vi "Quick Load WAV.vi"(8 "error in":errorcluster, 11 "Data":u8[](array[numeric])) -> (0 "error out":errorcluster, 3 "Chunk Pointer":u32 format="%.0x")   [LabVIEW 2014, in "LibSDL2_Mixer.lvlib"]
uses:
  LibSDL2_Mixer.lvlib
  LibSDL2 Wrapper/DLL/SDL2_mixer.dll
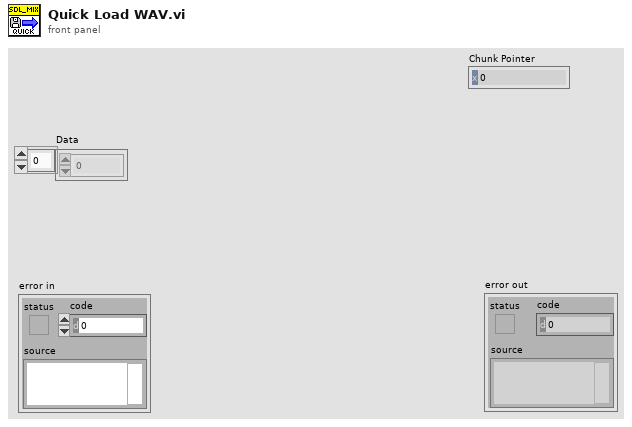
[diagram p1: front panel]
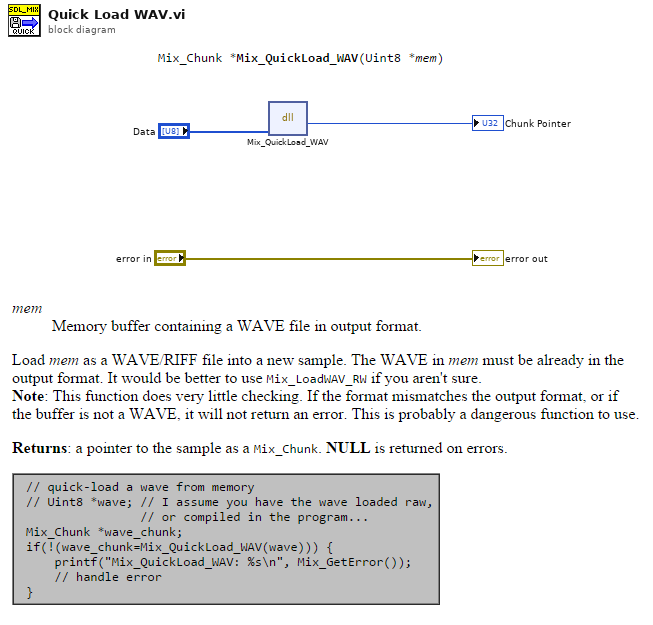
[diagram p0: block diagram]
diagram:
  n1 = dll-call lib="C:/dev/PGS/LabSDL2/Source/Libraries/LibSDL2 Wrapper/DLL/SDL2_mixer.dll" fn="Mix_QuickLoad_WAV"("mem"="Data") -> ("return type"=→"Chunk Pointer":u32)  [unwired: 4 in, 2 out]
  "error out" <- "error in"
